vi "niDTS BT Tx Test UTIL BT TX Parameters to EDR Parameters.vi"(7 "BT Tx Input Parameters":T10={"Channel"=0, "Data Rate "=1, "Dut Tx Power"=0.0, "External Attenuation (dB)"=[0.0, 0.0, 0.0, 0.0], "Auto Level"=FALSE, "Packet type"=enum."DH1", "Payload Pattern"=enum."PN9", "Burst Sync"=enum."PREamble", "BD ADDRESS"=0, "Packet Length, bytes"=37, "ModAcc Measurement Paramaters"={"ModAcc Enable"=FALSE, "CFO Enable"=FALSE, "Character Select"=enum."DF1", "Averages"=1, "Averaging Mode"=enum."RMS", "Measurement Length"=-1, "Measurement Offset"=0}, "OBW Measurement Parameters"={"OBW Enable"=FALSE, "OBW Averages"=1, "Averaging Type"=enum."RMS", "Measurement Interval Mode"=enum."AUTO", "Measurement Interval Length (sec)"=0.005}, "TXP Measurement Parameters"={"TXP Power Enable"=FALSE, "TXP Averages"=1, "Averaging Type"=enum."RMS"}, "IBE  Measurement Parameters"={"IBE Enable"=FALSE, "IBE Averages"=1, "Averaging Type"=enum."RMS", "Numbe of Channels"=11, "Channel Mode"=enum."Centered", "Measurement Interval Mode"=enum."AUTO", "Measurement Interval Length (sec)"=0.005}, "Trace Enable"=FALSE, "Trigger"={"MinQuietTimeDuration (sec)"=0.0001, "TriggerDelay (sec)"=0.0, "TriggerEdge"=enum."RISing", "TriggerSource"=enum."RF0", "TriggerThreshold (dB)"=-20.0, "TriggerTimeout (sec)"=10.0}} {"BD ADDRESS" max=16777215 format="%.0x"}) -> (8 "output cluster":T1={"Channel"=3, "Dut Tx Power  (dBm)"=0.0, "Auto Level"=FALSE, "External Attenuation (dB)"=0.0, "EDR Packet type"=enum."DH1", "Data Rate"=2, "Payload Data"=enum."PN9", "Burst Sync"=enum."PREamble", "Packet Length, bytes"=-1, "BD ADDRESS"="", "Trace Enable"=FALSE, "EDR ModAcc Measurement"={"DEVM Enable"=FALSE, "Averages"=1, "Averaging Mode"=enum."RMS", "Measurement Duration (bytes)"=-1, "Measurement Offset (bytes)"=0}, "TXP Measurement"={"TXP Power Enable"=FALSE, "TXP Averages"=1, "Averaging Type"=enum."RMS"}, "IBE  Measurement"={"IBE Enable"=FALSE, "IBE Averages"=1, "Averaging Type"=enum."RMS", "Numbe of Channels"=11, "Channel Mode"=enum."Centered", "Measurement Interval Mode"=enum."AUTO", "Measurement Interval Length (sec)"=0.005}, "Trigger"={"MinQuietTimeDuration (sec)"=0.0001, "TriggerDelay (sec)"=0.0, "TriggerEdge"=enum."RISing", "TriggerSource"=enum."RF0", "TriggerThreshold (dB)"=20.0, "TriggerTimeout (sec)"=10.0}} {"Trigger"."MinQuietTimeDuration (sec)" format="%#_6p"; "Data Rate" min=2 max=3 step=1})   [LabVIEW 2014, in "niDTS BT.lvlib"]
uses:
  niDTS BT.lvlib
  Tx Test/Includes/niDTS BT Tx Test INC Parameters.ctl
  Includes/niDTS BT INC Packet Type.ctl
  Tx Test/Includes/niDTS BT Tx Test INC BD Payload Data.ctl
  Tx Test/Includes/niDTS BT Tx Test INC Modulation Characteristics.ctl
  Includes/niDTS BT INC OBW Measurement Parameters.ctl
  Includes/niDTS BT INC TXP Measurement Parameters.ctl
  Includes/niDTS BT INC EDR IBE Measurement Parameters.ctl
  Includes/niDTS BT DUT INC Trigger.ctl
  Includes/niDTS BT EDR Tx Test INC Parameters.ctl
  Includes/niDTS BT INC EDR Packet Type.ctl
  Includes/niDTS BT INC EDR Data Rate.ctl
  Includes/niDTS BT INC EDR Burst Sync.ctl
  Includes/niDTS BT INC EDR ModAcc Measurement Parameters.ctl
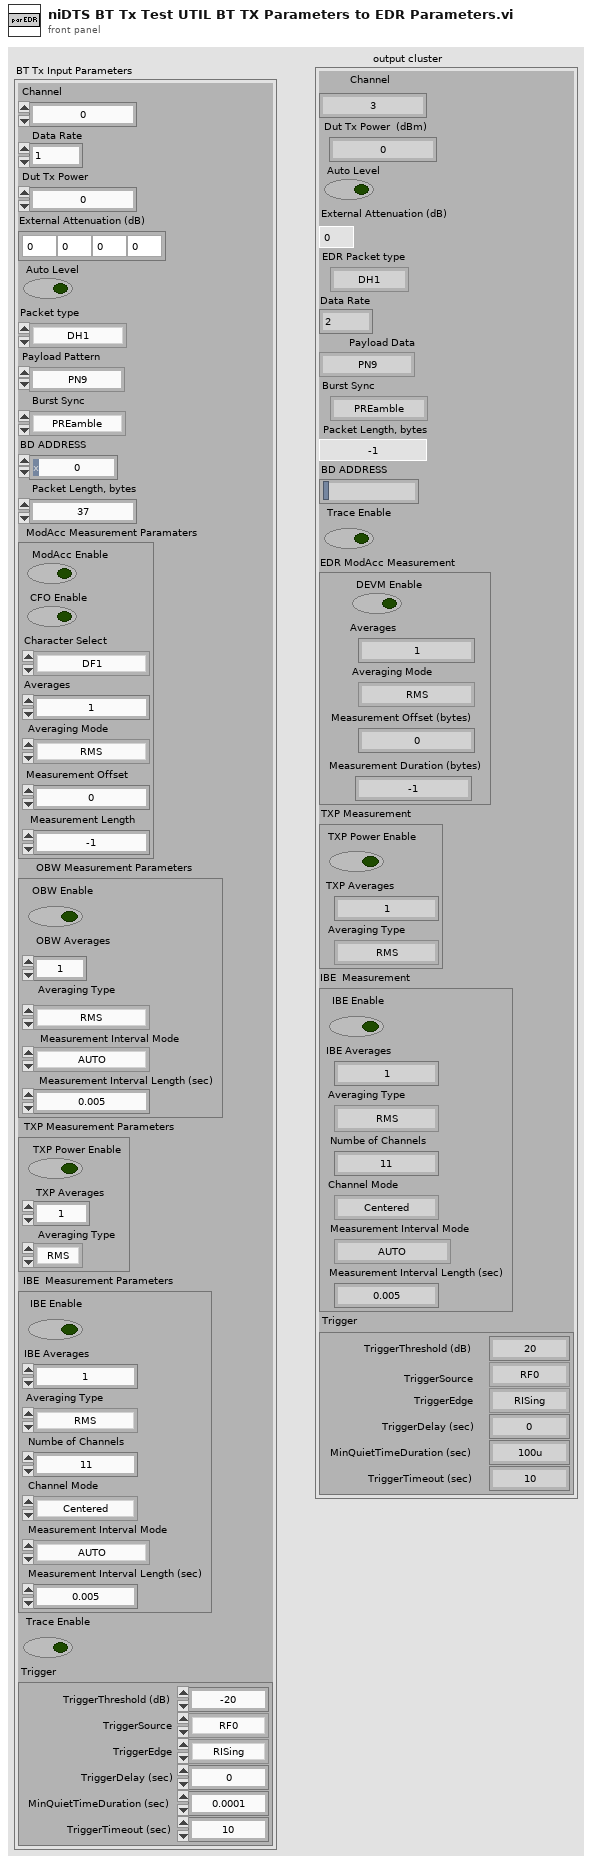
[diagram p1: front panel]
types:
  T1 = typedef "niDTS BT.lvlib/niDTS BT EDR Tx Test INC Parameters.ctl" = cluster{"Channel":i32, "Dut Tx Power  (dBm)":dbl, "Auto Level":bool, "External Attenuation (dB)":dbl, "EDR Packet type":T2, "Data Rate":T3, "Payload Data":T4, "Burst Sync":T5, "Packet Length, bytes":i32, "BD ADDRESS":string, "Trace Enable":bool, "EDR ModAcc Measurement":T6, "TXP Measurement":T7, "IBE  Measurement":T8, "Trigger":T9}
  T2 = typedef "niDTS BT.lvlib/niDTS BT INC EDR Packet Type.ctl" = enum16{"NULL", "POLL", "FHS", "DM1", "DH1", "HV1", "HV2", "HV3", "EV3", "DV", "AUX1", "DM3", "DH3", "EV4", "EV5", "DM5", "DH5"}
  T3 = typedef "niDTS BT.lvlib/niDTS BT INC EDR Data Rate.ctl" = i32
  T4 = typedef "niDTS BT.lvlib/niDTS BT Tx Test INC BD Payload Data.ctl" = enum16{"0", "1", "01", "00001111", "PN9", "AUTO"}
  T5 = typedef "niDTS BT.lvlib/niDTS BT INC EDR Burst Sync.ctl" = enum16{"NONE", "PREamble"}
  T6 = typedef "niDTS BT.lvlib/niDTS BT INC EDR ModAcc Measurement Parameters.ctl" = cluster{"DEVM Enable":bool, "Averages":i32, "Averaging Mode":enum16{"RMS", "LOG", "SCALAR", "MAX", "MIN", "VECTOR"}, "Measurement Duration (bytes)":i32, "Measurement Offset (bytes)":i32}
  T7 = typedef "niDTS BT.lvlib/niDTS BT INC TXP Measurement Parameters.ctl" = cluster{"TXP Power Enable":bool, "TXP Averages":i32, "Averaging Type":enum16{"RMS", "LOG", "SCALAR", "MAX", "MIN"}}
  T8 = typedef "niDTS BT.lvlib/niDTS BT INC EDR IBE Measurement Parameters.ctl" = cluster{"IBE Enable":bool, "IBE Averages":i32, "Averaging Type":enum16{"RMS", "LOG", "SCALAR", "MAX", "MIN", "VECTOR"}, "Numbe of Channels":i32, "Channel Mode":enum16{"InBand", "Centered"}, "Measurement Interval Mode":enum16{"AUTO", "MANUAL"}, "Measurement Interval Length (sec)":dbl}
  T9 = typedef "niDTS BT.lvlib/niDTS BT DUT INC Trigger.ctl" = cluster{"MinQuietTimeDuration (sec)":dbl, "TriggerDelay (sec)":dbl, "TriggerEdge":enum16{"RISing", "FALLing"}, "TriggerSource":enum16{"IMMediate", "RF0", "PFI0", "PFI1", "RTS0", "RTS1", "RTS2", "RTS3", "RTS4", "RTS5", "RTS6", "RTS7", "PXIStar", "SOFT"}, "TriggerThreshold (dB)":dbl, "TriggerTimeout (sec)":dbl}
  T10 = typedef "niDTS BT.lvlib/niDTS BT Tx Test INC Parameters.ctl" = cluster{"Channel":i32, "Data Rate ":i32, "Dut Tx Power":dbl, "External Attenuation (dB)":dbl[], "Auto Level":bool, "Packet type":T11, "Payload Pattern":T4, "Burst Sync":enum16{"NONE", "PREamble"}, "BD ADDRESS":u32, "Packet Length, bytes":i32, "ModAcc Measurement Paramaters":cluster{"ModAcc Enable":bool, "CFO Enable":bool, "Character Select":T12, "Averages":i32, "Averaging Mode":enum16{"RMS", "LOG", "SCALAR", "MAX", "MIN", "VECTOR"}, "Measurement Length":i32, "Measurement Offset":i32}, "OBW Measurement Parameters":T13, "TXP Measurement Parameters":T7, "IBE  Measurement Parameters":T8, "Trace Enable":bool, "Trigger":T9}
  T11 = typedef "niDTS BT.lvlib/niDTS BT INC Packet Type.ctl" = enum16{"NULL", "POLL", "FHS", "DM1", "DH1", "HV1", "HV2", "HV3", "EV3", "DV", "AUX1", "DM3", "DH3", "EV4", "EV5", "DM5", "DH5", "LE-TP"}
  T12 = typedef "niDTS BT.lvlib/niDTS BT Tx Test INC Modulation Characteristics.ctl" = enum16{"DF1", "DF2", "BOTH"}
  T13 = typedef "niDTS BT.lvlib/niDTS BT INC OBW Measurement Parameters.ctl" = cluster{"OBW Enable":bool, "OBW Averages":i32, "Averaging Type":enum16{"RMS", "LOG", "SCALAR", "MAX", "MIN", "VECTOR"}, "Measurement Interval Mode":enum16{"AUTO", "MANUAL"}, "Measurement Interval Length (sec)":dbl}
  T14 = cluster{"ModAcc Enable":bool, "CFO Enable":bool, "Character Select":T12, "Averages":i32, "Averaging Mode":enum16{"RMS", "LOG", "SCALAR", "MAX", "MIN", "VECTOR"}, "Measurement Length":i32, "Measurement Offset":i32}
  T15 = enum16{"NULL", "POLL", "FHS", "DM1", "DH1", "HV1", "HV2", "HV3", "EV3", "DV", "AUX1", "DM3", "DH3", "EV4", "EV5", "DM5", "DH5"}
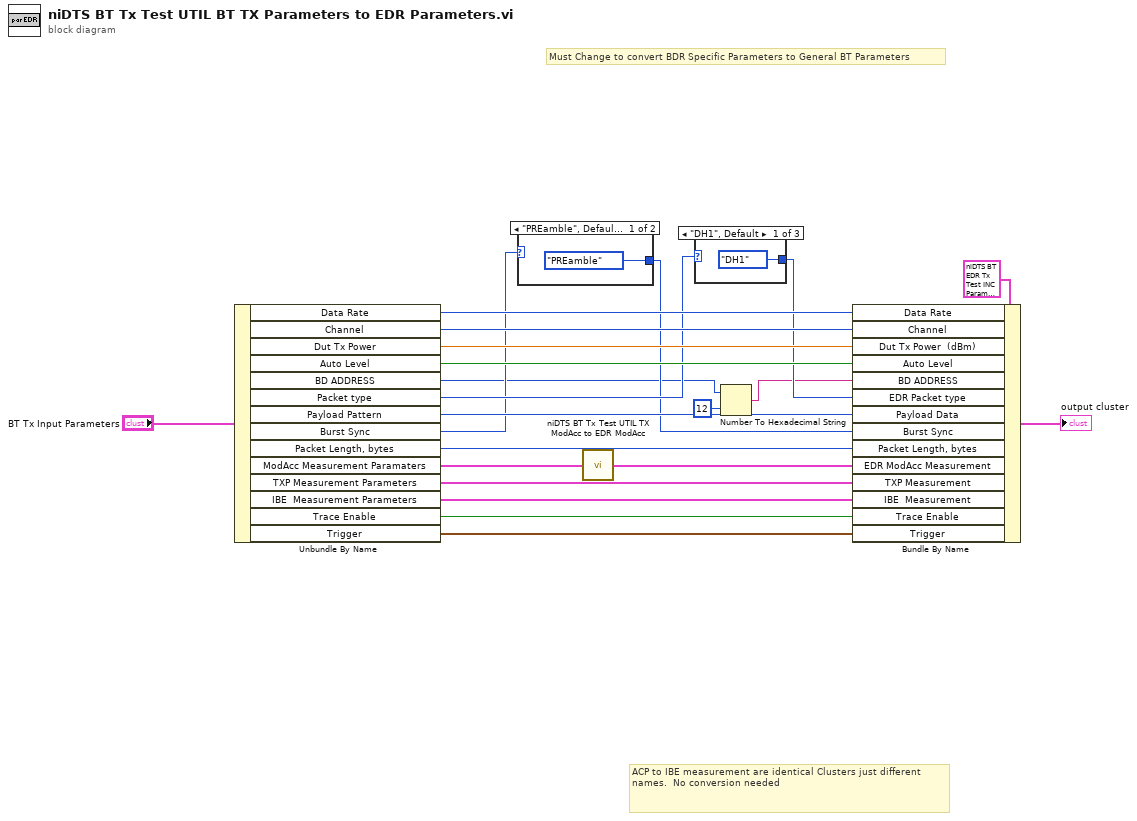
[diagram p0: block diagram]
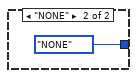
[diagram p2: hidden frame]
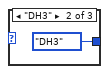
[diagram p3: hidden frame]
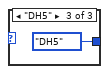
[diagram p4: hidden frame]
diagram:
  # "ACP to IBE measurement are identical Clusters just different names.  No conversion needed"
  # "Must Change to convert BDR Specific Parameters to General BT Parameters"
  n1 = Unbundle By Name("BT Tx Input Parameters") -> ("Data Rate"=w15:i32, "Channel"=w22:i32, "Dut Tx Power"=w21:dbl, "Auto Level"=w20:bool, "BD ADDRESS"=w4:u32, "Packet type"=w12:T11, "Payload Pattern"=w19:T4, "Burst Sync"=w10:enum16{"NONE", "PREamble"}, "Packet Length, bytes"=w6:i32, "ModAcc Measurement Paramaters"=w7:T14, "TXP Measurement Parameters"=w18:T7, "IBE  Measurement Parameters"=w13:T8, "Trace Enable"=w17:bool, "Trigger"=w16:T9)
  n2 = case shown="\"PREamble\", Default" w10 {
    tunnel: [niDTS_BT_INC_EDR_Burst_Sync."PREamble" ("Burst Sync") niDTS_BT_INC_EDR_Burst_Sync."NONE" ("Burst Sync")] -> w9
    frame "PREamble", Default {
    }
    frame "NONE" {
    }
  }
  n3 = call "niDTS BT Tx Test UTIL TX ModAcc to EDR ModAcc.vi"("ModAcc Measurement Paramaters in"=w7) -> ("ModAcc Measurement Paramaters"=w5:T6)  [unwired: 14 in]
  n4 = case shown="\"DH1\", Default" w12 {
    tunnel: [T15."DH1" T15."DH3" T15."DH5"] -> w11
    frame "DH1", Default {
    }
    frame "DH3" {
    }
    frame "DH5" {
    }
  }
  n5 = Number To Hexadecimal String(1:i16 12 ("width (-)"), 2:w4) -> (0:w2:string)
  n6 = Bundle By Name(cluster=T1 {"Channel"=3, "Dut Tx Power  (dBm)"=0.0, "Auto Level"=FALSE, "External Attenuation (dB)"=0.0, "EDR Packet type"=enum."DH1", "Data Rate"=2, "Payload Data"=enum."PN9", "Burst Sync"=enum."PREamble", "Packet Length, bytes"=-1, "BD ADDRESS"="", "Trace Enable"=FALSE, "EDR ModAcc Measurement"={"DEVM Enable"=FALSE, "Averages"=1, "Averaging Mode"=enum."RMS", "Measurement Duration (bytes)"=-1, "Measurement Offset (bytes)"=0}, "TXP Measurement"={"TXP Power Enable"=FALSE, "TXP Averages"=1, "Averaging Type"=enum."RMS"}, "IBE  Measurement"={"IBE Enable"=FALSE, "IBE Averages"=1, "Averaging Type"=enum."RMS", "Numbe of Channels"=11, "Channel Mode"=enum."Centered", "Measurement Interval Mode"=enum."AUTO", "Measurement Interval Length (sec)"=0.005}, "Trigger"={"MinQuietTimeDuration (sec)"=0.0001, "TriggerDelay (sec)"=0.0, "TriggerEdge"=enum."RISing", "TriggerSource"=enum."RF0", "TriggerThreshold (dB)"=20.0, "TriggerTimeout (sec)"=10.0}} ("EDR Tx Input Parameters"), "Data Rate"=w15, "Channel"=w22, "Dut Tx Power  (dBm)"=w21, "Auto Level"=w20, "BD ADDRESS"=w2, "EDR Packet type"=w11, "Payload Data"=w19, "Burst Sync"=w9, "Packet Length, bytes"=w6, "EDR ModAcc Measurement"=w5, "TXP Measurement"=w18, "IBE  Measurement"=w13, "Trace Enable"=w17, "Trigger"=w16) -> (→"output cluster":T1)
